vi "P4.vi"() -> ()   [LabVIEW 2021]
uses:
  <vilib>/LabVIEW Interface for Arduino/Type Defs/Board Type.ctl
  <vilib>/LabVIEW Interface for Arduino/Type Defs/Connection Type.ctl
  <vilib>/LabVIEW Interface for Arduino/Type Defs/Pin Mode.ctl
  <vilib>/LabVIEW Interface for Arduino/LabVIEW Interface for Arduino.lvlib
panel:
  in  "CERRAR PUERTO":bool
  out "Medido A0":dbl(knob) scale=0.0..5.0
  out "LED 8":bool
  in  "PIN 8":bool
  out "Salida":dbl(slide) scale=0.0..255.0
  in  "Valor Analógico":dbl(knob) scale=0.0..255.0
  # "Practica 4: Lectura y Escritura de Valores"
  # "Valor enviado a salida PWM pin 3"
  # "Control salida digital pin 8"
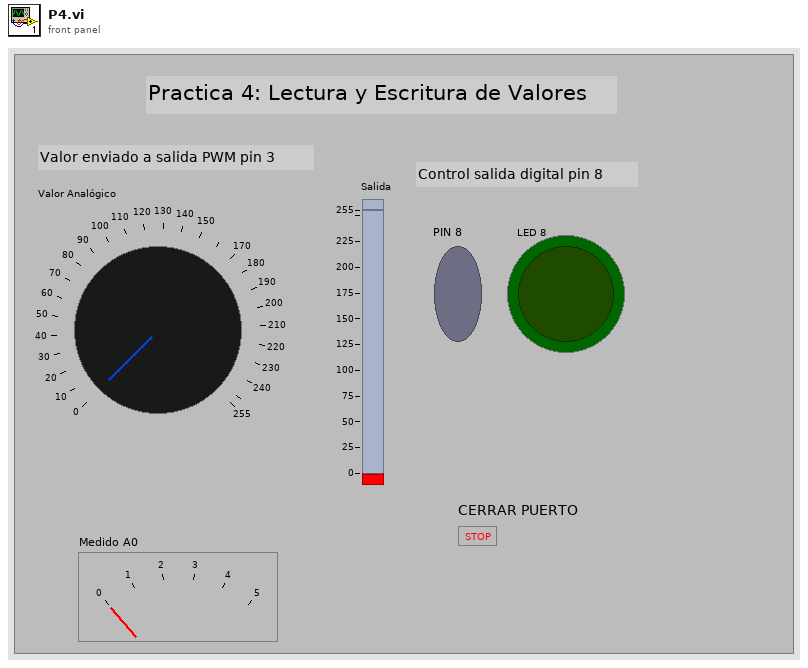
[diagram p1: front panel]
types:
  T1 = typedef "LabVIEW Interface for Arduino.lvlib/Pin Mode.ctl" = enum8{"Input", "Output"}
  T2 = typedef "LabVIEW Interface for Arduino.lvlib/Connection Type.ctl" = enum8{"USB / Serial", "XBEE", "BlueSmirf (Bluetooth)"}
  T3 = typedef "LabVIEW Interface for Arduino.lvlib/Board Type.ctl" = enum16{"Uno", "Dimuelanove w/Atmega 328", "Mega 2560"}
  T4 = typedef "LabVIEW Interface for Arduino.lvlib/Arduino Resource.ctl" = cluster{"VISA resource":refnum<visa-resource-name>, "Board Type":T3, "Connection Type":enum8{"USB / Serial"}, "Bytes Per Packet (15)":u8}
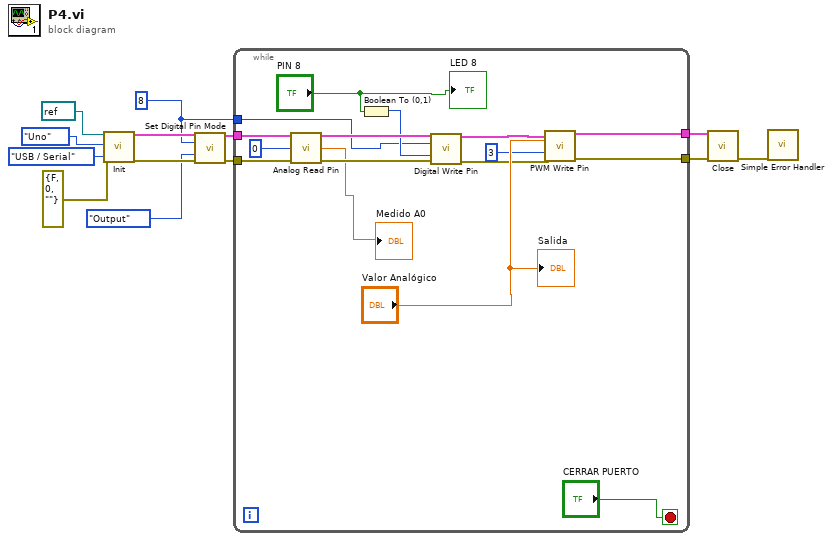
[diagram p0: block diagram]
diagram:
  w4 = u8 8 ("Digital I/O Pin")
  n1 = call <vilib>:"Init.vi"("VISA resource"=refnum<visa-resource-name> refnum, "Board Type (Uno)"=Board_Type."Uno", "Connection Type (USB/Serial)"=Connection_Type."USB / Serial", "error in"=errorcluster {"status"=FALSE, "code"=0, "source"=""}) -> ("Arduino Resource"=w9:T4, "error out"=w8:errorcluster)  [unwired: 14 in]
  n2 = call <vilib>:"Set Digital Pin Mode.vi"("Arduino Resource"=w9, "Digital I/O Pin"=w4, "Pin Mode (Input)"=Pin_Mode."Output", "error in"=w8) -> ("Arduino Resource"=w6:T4, "error out"=w5:errorcluster)  [unwired: 10 in]
  n3 = while {
    tunnel: w6 -> [w27]
    tunnel: w5 -> [w26]
    tunnel: w4 -> [w18]
    tunnel: [w23] -> w3
    tunnel: [w22] -> w2
    stop <- "CERRAR PUERTO" stop-if-true
    n4 = call <vilib>:"Analog Read Pin.vi"("Arduino Resource"=w27, "Analog Input Pin (0)"=u8 0, "error in"=w26) -> ("Arduino Resource"=w21:T4, "Voltage"=→"Medido A0":dbl, "error out"=w20:errorcluster)  [unwired: 10 in]
    n5 = Boolean To (0,1)(Boolean="PIN 8") -> (0, 1=w19:i16)
    n6 = call <vilib>:"Digital Write Pin.vi"("Arduino Resource"=w21, "Digital I/O Pin (0)"=w18, "Value (0)"=w19, "error in"=w20) -> ("Arduino Resource"=w16:T4, "error out"=w15:errorcluster)  [unwired: 10 in]
    n7 = call <vilib>:"PWM Write Pin.vi"("Arduino Resource"=w16, "Duty Cycle (0 - 255)"="Valor Analógico", "PWM Pin (3)"=u8 3, "error in"=w15) -> ("Arduino Resource"=w23:T4, "error out"=w22:errorcluster)  [unwired: 10 in]
    "Salida" <- "Valor Analógico"
    "LED 8" <- "PIN 8"
  }
  n8 = call <vilib>:"Close.vi"("Arduino Resource"=w3, "error in"=w2) -> ("error out"=w1:errorcluster)  [unwired: 13 in]
  n9 = call <vilib>:"Simple Error Handler.vi"("error in (no error)"=w1) -> ()  [unwired: 4 in, 5 out]
